vi "Get Plot Metadata.vi"(0 "Model?":bool, 5 "Row Number":i32[](array[numeric]), 7 "Source Location":i32[](array[numeric]), 9 "UVW":i32[](array[numeric]), 11 "Lower Upper":i32[](array[numeric]), 12 "Interation number":i32) -> (1 "Wind Direction":dbl format="%0.2f", 3 "Lower upper":string[][](array[string]), 4 "Locations":string[][](array[string]), 6 "UVW":string[][](array[string]), 8 "Source Locations":string[][](array[string]), 10 "Max Min array":dbl[][](array[numeric]), 13 "Raw Data Filenames":string[](array[string]), 15 "Stl Filename":string)   [LabVIEW 2021]
uses:
  Anemometry/Anemometry Sub Vis/Data_plotting_vis/Results_plotter_Global.vi
  <vilib>/Analysis/NI_AALBase.lvlib
  RFP_Table_Global.vi
  <vilib>/Analysis/baseanly.llb/Mean (DBL).vi
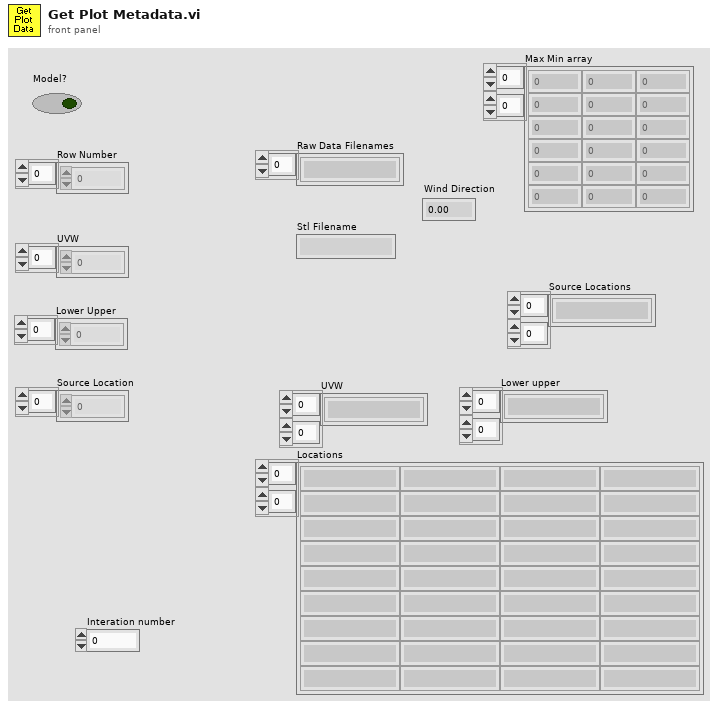
[diagram p1: front panel]
types:
  T1 = enum16{"To Traverse Coordinates", "To User Coordinates"}
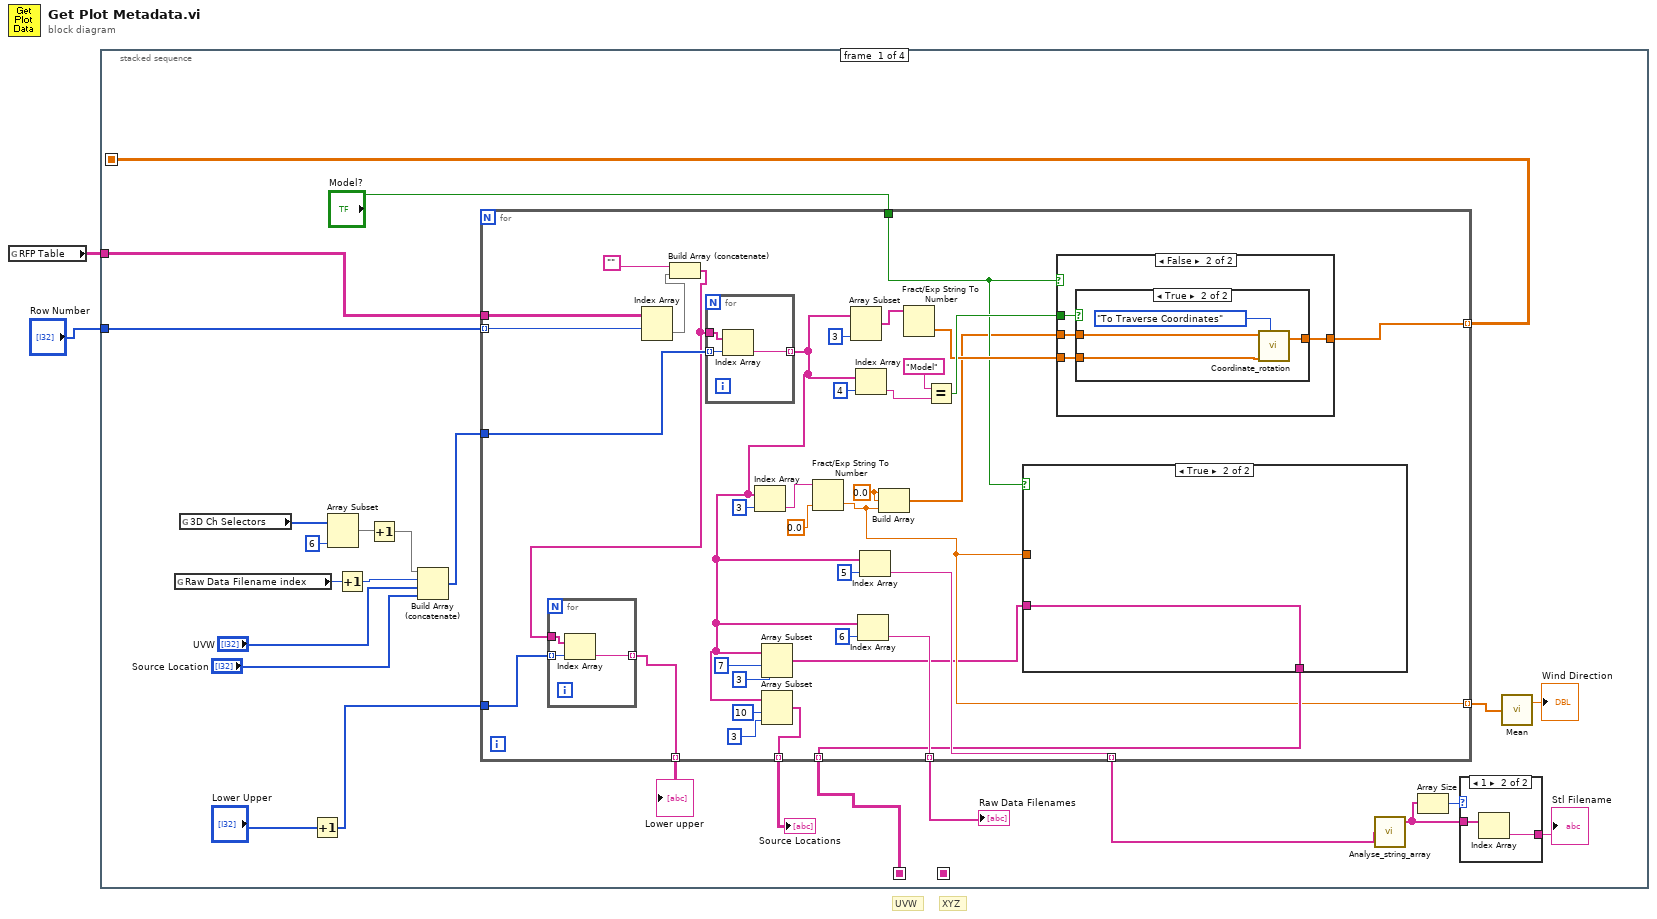
[diagram p0: block diagram]
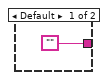
[diagram p2: hidden frame]
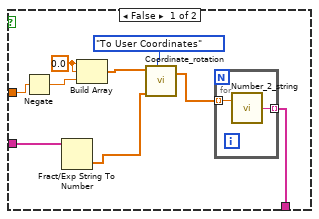
[diagram p3: hidden frame]
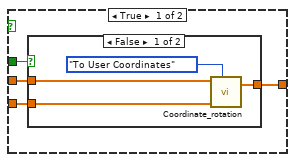
[diagram p4: hidden frame]
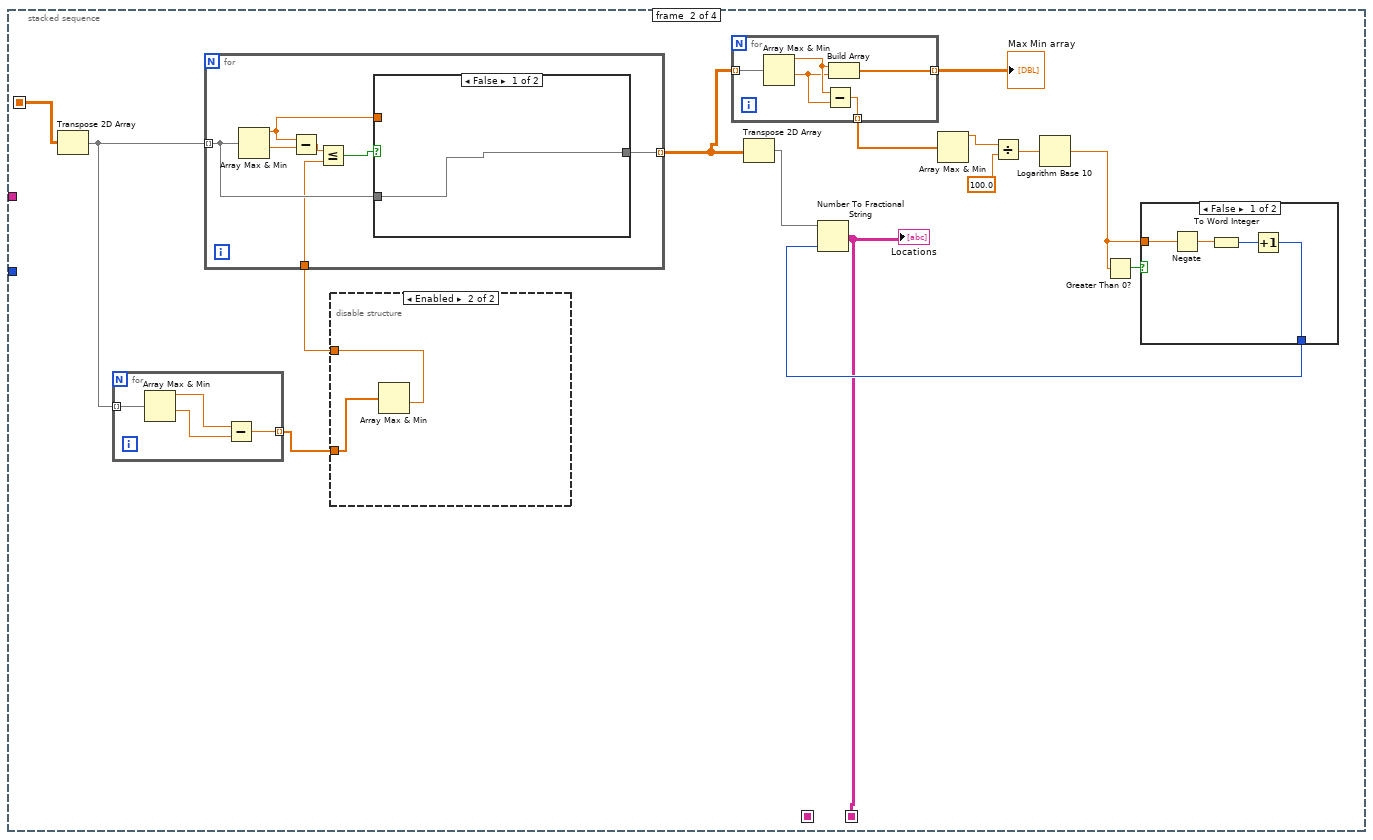
[diagram p7: hidden frame]
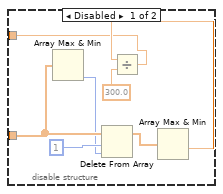
[diagram p8: hidden frame]
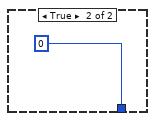
[diagram p9: hidden frame]
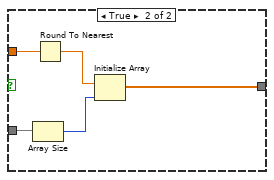
[diagram p10: hidden frame]
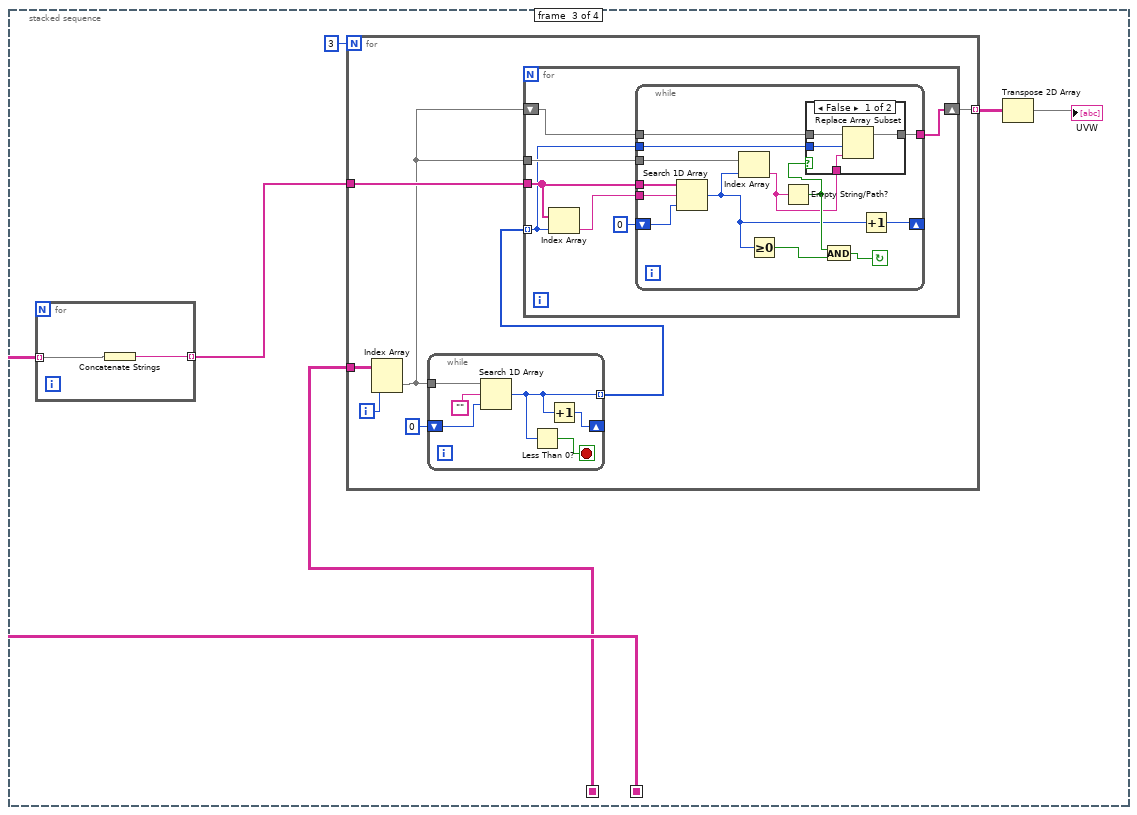
[diagram p11: hidden frame]
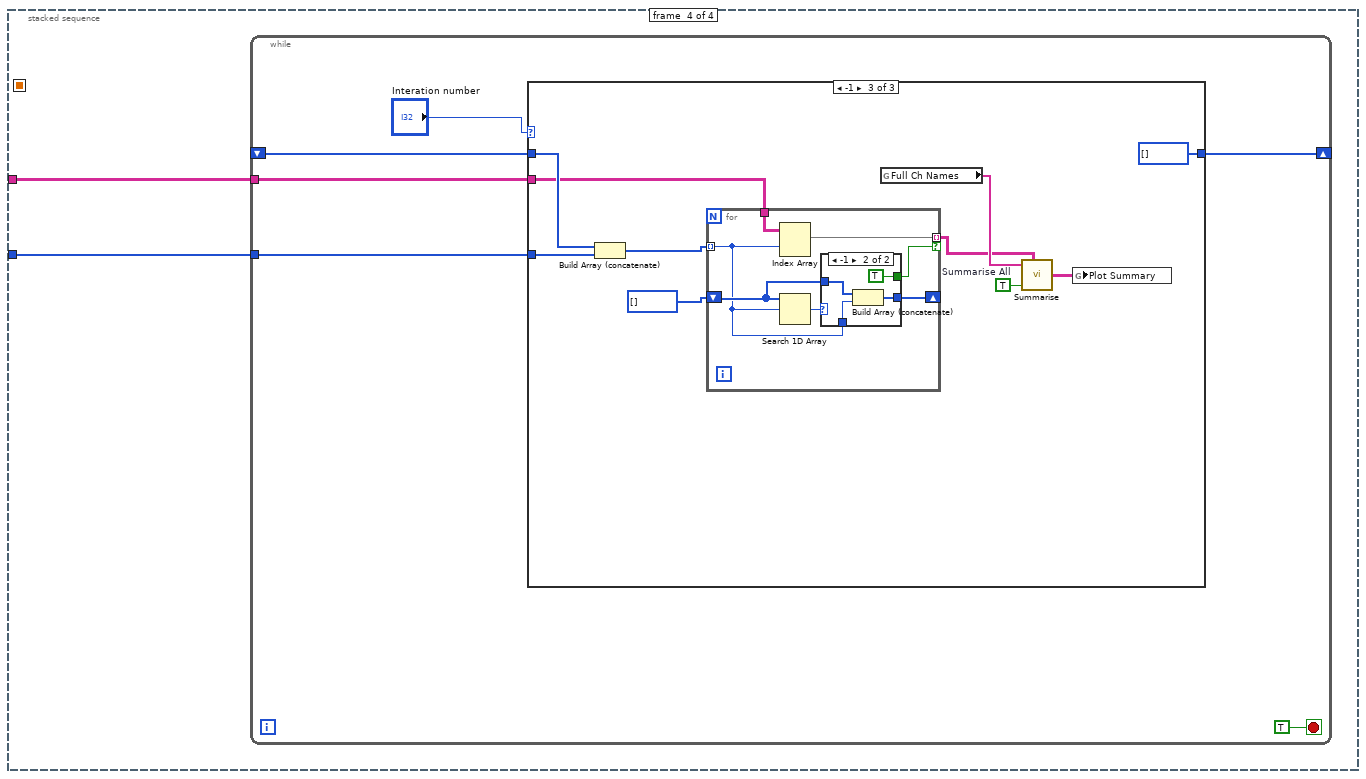
[diagram p13: hidden frame]
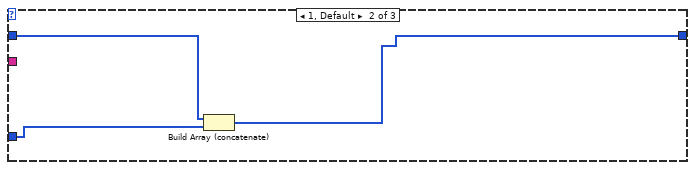
[diagram p15: hidden frame]
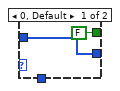
[diagram p16: hidden frame]
diagram:
  # "XYZ"
  # "UVW"
  n1 = global read "RFP_Table_Global.vi" "RFP Table"() -> (w2:string[][])
  n2 = stacked-sequence {
    seq-local: [w24 _ _ _] -> [_ w105 _ _]
    seq-local: [w5 _ _ _] -> [_ _ w156 _]
    seq-local: [_ w102 _ _] -> [_ _ w158 _]
    tunnel: w2 -> [w4 _ _ w199]
    tunnel: "Row Number" -> [w3 _ _ w200]
    frame #0 {
      n3 = global read "Results_plotter_Global.vi" "Raw Data Filename index"() -> (w22:i32)
      n4 = global read "Results_plotter_Global.vi" "3D Ch Selectors"() -> (w26:i32[])
      n5 = Increment(x="Lower Upper") -> (x+1=w11:i32[])
      n6 = Array Subset(array=w26, length=6) -> (w7:i32[])  [unwired: 1 in]
      n7 = Increment(x=w22) -> (x+1=w17:i32)
      n8 = Increment(x=w7) -> (x+1=w6:i32[])
      n9 = Build Array (concatenate)(w6, w17, "UVW", "Source Location") -> (w23:i32[])
      n10 = for {
        tunnel: w3 -> [w65] mode=indexing
        tunnel: w23 -> [w64]
        tunnel: "Model?" -> [w46]
        tunnel: [w54] -> w24 mode=indexing
        tunnel: [w44] -> w5 mode=indexing
        tunnel: [w49] -> w18 mode=indexing
        tunnel: [w47] -> w15 mode=indexing
        tunnel: [w43] -> w14 mode=indexing
        tunnel: w11 -> [w41]
        tunnel: [w40] -> w10 mode=indexing
        tunnel: [w34] -> w8 mode=indexing
        tunnel: w4 -> [w31]
        w57 = 0.0 ("element")
        n11 = Index Array(array=w31, index (row)=w65) -> (element=w51:string[])  [unwired: 1 in]
        n12 = Build Array (concatenate)("", w51) -> (w42:string[])
        n13 = for {
          tunnel: w41 -> [w68] mode=indexing
          tunnel: w42 -> [w67]
          tunnel: [w66] -> w40 mode=indexing
          n14 = Index Array(array=w67, index=w68) -> (element=w66:string)
        }
        n15 = for {
          tunnel: w64 -> [w101] mode=indexing
          tunnel: w42 -> [w100]
          tunnel: [w99] -> w37 mode=indexing
          n16 = Index Array(array=w100, index=w101) -> (element=w99:string)
        }
        n17 = Index Array(array=w37, index=3) -> (element=w56:string)
        n18 = Array Subset(array=w37, index=7, length=3) -> (w38:string[])
        n19 = Array Subset(array=w37, index=10, length=3) -> (w34:string[])
        n20 = Fract/Exp String To Number(string=w56, default (0 dbl)=0.0 ("default (0 DBL)")) -> (number=w43:dbl)  [unwired: 2 in, 1 out]
        n21 = Array Subset(array=w37, length=3) -> (w61:string[])  [unwired: 1 in]
        n22 = Index Array(array=w37, index=4) -> (element=w60:string)
        n23 = Index Array(array=w37, index=6) -> (element=w47:string)
        n24 = Index Array(array=w37, index=5) -> (element=w49:string)
        n25 = Build Array(w57, w57, w43) -> (w45:dbl[])
        n26 = Fract/Exp String To Number(string=w61) -> (number=w53:dbl[])  [unwired: 3 in, 1 out]
        n27 = Equal?(x="Model", y=w60) -> (x = y?=w55:bool)
        n28 = case shown="True" w46 {
          tunnel: [w76 w80] -> w44
          tunnel: w38 -> [w75 w80]
          tunnel: w43 -> [w69 _]
          frame False {
            w72 = 0.0 ("element")
            n29 = Negate(x=w69) -> (-x=w70:dbl)
            n30 = Fract/Exp String To Number(string=w75) -> (number=w74:dbl[])  [unwired: 3 in, 1 out]
            n31 = Build Array(w72, w72, w70) -> (w71:dbl[])
            n32 = call "Coordinate_rotation.vi"("Roll-Pitch-Yaw"=w71, "Input Position"=w74, "Mode"=T1."To User Coordinates") -> ("Output Position"=w73:sgl[])  [unwired: 2 in, 1 out]
            n33 = for {
              tunnel: w73 -> [w79] mode=indexing
              tunnel: [w78] -> w76 mode=indexing
              n34 = call "Number_2_string.vi"("number"=w79) -> ("String"=w78:string)  [unwired: 1 in]
            }
          }
          frame True {
          }
        }
        n35 = case shown="False" w46 {
          tunnel: w55 -> [w84 w93]
          tunnel: [w83 w92] -> w54
          tunnel: w53 -> [w82 w91]
          tunnel: w45 -> [w81 w90]
          frame True {
            n36 = case shown="False" w84 {
              tunnel: [w85 w89] -> w83
              tunnel: w82 -> [w87 w89]
              tunnel: w81 -> [w86 _]
              frame False {
                n37 = call "Coordinate_rotation.vi"("Roll-Pitch-Yaw"=w86, "Input Position"=w87, "Mode"=T1."To User Coordinates") -> ("Output Position"=w85:sgl[])  [unwired: 2 in, 1 out]
              }
              frame True {
              }
            }
          }
          frame False {
            n38 = case shown="True" w93 {
              tunnel: [w94 w97] -> w92
              tunnel: w91 -> [w94 w98]
              tunnel: w90 -> [_ w96]
              frame False {
              }
              frame True {
                n39 = call "Coordinate_rotation.vi"("Roll-Pitch-Yaw"=w96, "Input Position"=w98, "Mode"=T1."To Traverse Coordinates") -> ("Output Position"=w97:sgl[])  [unwired: 2 in, 1 out]
              }
            }
          }
        }
      }
      "Raw Data Filenames" <- w15
      "Lower upper" <- w10
      "Source Locations" <- w8
      n40 = call "Analyse_string_array.vi"("String array"=w18) -> ("Unique strings"=w20:string[])  [unwired: 1 in, 1 out]
      n41 = Array Size(array=w20) -> (size(s)=w21:i32)
      n42 = case shown="1" w21 {
        tunnel: w20 -> [_ w30]
        tunnel: ["" w29] -> w19
        frame Default {
        }
        frame 1 {
          n43 = Index Array(array=w30) -> (element=w29:string)  [unwired: 1 in]
        }
      }
      "Stl Filename" <- w19
      n44 = call-poly <vilib>:"Mean.vi"("X"=w14) -> ("mean"=→"Wind Direction":dbl)  [unwired: 1 out]
    }
    frame #1 {
      n45 = Transpose 2D Array(2D array=w105) -> (transposed array=w106:dbl[][])
      n46 = for {
        tunnel: w106 -> [w129] mode=indexing
        tunnel: [w127] -> w104 mode=indexing
        n47 = Array Max & Min(array=w129) -> (max value=w128:dbl, min value=w126:dbl)  [unwired: 2 out]
        n48 = Subtract(x=w128, y=w126) -> (x-y=w127:dbl)
      }
      n49 = disable-structure shown="Enabled" {
        disable-tunnel: w104 -> [w122 w125]
        disable-tunnel: [w118 w124] -> w103
        frame Disabled {
          n50 = Array Max & Min(array=w122) -> (min index (indices)=w117:i32)  [unwired: 3 out]
          n51 = Delete From Array(array=w122, length=1, index=w117) -> (array with subset deleted=w119:dbl[])  [unwired: 1 out]
          n52 = Array Max & Min(array=w119) -> (min value=w120:dbl)  [unwired: 3 out]
          n53 = Divide(x=w120, y=300.0) -> (x/y=w118:dbl)
        }
        frame Enabled {
          n54 = Array Max & Min(array=w125) -> (min value=w124:dbl)  [unwired: 3 out]
        }
      }
      n55 = for {
        tunnel: w106 -> [w143] mode=indexing
        tunnel: [w142] -> w116 mode=indexing
        tunnel: w103 -> [w141]
        n56 = Array Max & Min(array=w143) -> (max value=w144:dbl, min value=w146:dbl)  [unwired: 2 out]
        n57 = Subtract(x=w144, y=w146) -> (x-y=w145:dbl)
        n58 = Less Or Equal?(x=w145, y=w141) -> (x <= y?=w140:bool)
        n59 = case shown="False" w140 {
          tunnel: w144 -> [_ w152]
          tunnel: w143 -> [w147 w151]
          tunnel: [w147 w148] -> w142
          frame False {
          }
          frame True {
            n60 = Array Size(array=w151) -> (size(s)=w150:i32)
            n61 = Round To Nearest(number=w152) -> (nearest integer value=w149:dbl)
            n62 = Initialize Array(w149, w150) -> (w148:dbl[])
          }
        }
      }
      n63 = for {
        tunnel: w116 -> [w139] mode=indexing
        tunnel: [w138] -> w115 mode=indexing
        tunnel: [w135] -> w113 mode=indexing
        n64 = Array Max & Min(array=w139) -> (max value=w137:dbl, min value=w136:dbl)  [unwired: 2 out]
        n65 = Subtract(x=w137, y=w136) -> (x-y=w135:dbl)
        n66 = Build Array(w137, w136) -> (w138:dbl[])
      }
      "Max Min array" <- w115
      n67 = Transpose 2D Array(2D array=w116) -> (transposed array=w114:dbl[][])
      n68 = Array Max & Min(array=w113) -> (max value=w112:dbl)  [unwired: 3 out]
      n69 = Divide(x=w112, y=100.0) -> (x/y=w110:dbl)
      n70 = Logarithm Base 10(1:w110) -> (0:w108:dbl)
      n71 = Greater Than 0?(x=w108) -> (x > 0?=w109:bool)
      n72 = case shown="False" w109 {
        tunnel: w108 -> [w133 _]
        tunnel: [w130 i16 0 ("precision (6)")] -> w107
        frame False {
          n73 = Negate(x=w133) -> (-x=w132:dbl)
          n74 = To Word Integer(number=w132) -> (16bit integer=w131:i16)
          n75 = Increment(x=w131) -> (x+1=w130:i16)
        }
        frame True {
        }
      }
      n76 = Number To Fractional String(number=w114, precision (6)=w107) -> (F-format string=w102:string[][])  [unwired: 2 in]
      "Locations" <- w102
    }
    frame #2 {
      n77 = for {
        tunnel: w158 -> [w198] mode=indexing
        tunnel: [w197] -> w157 mode=indexing
        n78 = Concatenate Strings(w198) -> (w197:string)
      }
      n79 = for {
        N: 3 -> [_]
        tunnel: w157 -> [w161]
        tunnel: w156 -> [w165]
        tunnel: [w159] -> w154 mode=indexing
        i -> [w164]
        n80 = Index Array(array=w165, index (col)=w164) -> (element=w160:string[])  [unwired: 1 in]
        n81 = while {
          tunnel: w160 -> [w171]
          shift-right: [w166] -> _
          shift-left: 0 ("index of element") -> [w169]
          tunnel: [w167] -> w162 mode=indexing
          stop <- w168 stop-if-true
          n82 = Search 1D Array(1D array=w171, element="", start index (0)=w169) -> (index of element=w167:i32)
          n83 = Less Than 0?(x=w167) -> (x < 0?=w168:bool)
          n84 = Increment(x=w167) -> (x+1=w166:i32)
        }
        n85 = for {
          tunnel: w161 -> [w178]
          tunnel: w162 -> [w172] mode=indexing
          tunnel: w160 -> [w175]
          shift-right: [w173] -> w159
          shift-left: w160 -> [w174]
          n86 = Index Array(array=w178, index=w172) -> (element=w177:string)
          n87 = while {
            tunnel: w178 -> [w191]
            tunnel: w177 -> [w190]
            shift-right: [w179] -> _
            shift-left: 0 ("index of element") -> [w189]
            tunnel: w175 -> [w188]
            tunnel: w174 -> [w184]
            tunnel: [w183] -> w173
            tunnel: w172 -> [w181]
            stop <- w186 continue-if-true
            n88 = Search 1D Array(1D array=w191, element=w190, start index (0)=w189) -> (index of element=w180:i32)
            n89 = Index Array(array=w188, index=w180) -> (element=w182:string)
            n90 = Greater Or Equal To 0?(x=w180) -> (x >= 0?=w187:bool)
            n91 = Empty String/Path?(string/path=w182) -> (empty?=w185:bool)
            n92 = case shown="False" w185 {
              tunnel: w184 -> [w195 w196]
              tunnel: [w194 w196] -> w183
              tunnel: w181 -> [w193 _]
              tunnel: w182 -> [w192 _]
              frame False {
                n93 = Replace Array Subset(array=w195, new element=w192, index=w193) -> (w194:string[])
              }
              frame True {
              }
            }
            n94 = And(x=w185, y=w187) -> (x .and. y?=w186:bool)
            n95 = Increment(x=w180) -> (x+1=w179:i32)
          }
        }
      }
      n96 = Transpose 2D Array(2D array=w154) -> (transposed array=→"UVW":string[][])
    }
    frame #3 {
      n97 = while {
        shift-right: [w205] -> _
        shift-left: _ -> [w203]
        tunnel: w200 -> [w204]
        tunnel: w199 -> [w201]
        stop <- TRUE stop-if-true
        n98 = case shown="-1" "Interation number" {
          tunnel: [w207 w208 i32[] [] ("Row Number")] -> w205
          tunnel: w204 -> [w207 w210 w220]
          tunnel: w203 -> [_ w209 w219]
          tunnel: w201 -> [_ _ w216]
          frame 0 {
          }
          frame 1, Default {
            n99 = Build Array (concatenate)(w209, w210) -> (w208:i32[])
          }
          frame -1 {
            w218 = TRUE  # Summarise All
            n100 = Build Array (concatenate)(w219, w220) -> (w215:i32[])
            n101 = for {
              tunnel: w216 -> [w227]
              tunnel: [w226] -> w212 mode=indexing if=w222
              tunnel: w215 -> [w221] mode=indexing
              shift-right: [w224] -> _
              shift-left: i32[] [] -> [w223]
              n102 = Index Array(array=w227, index (row)=w221) -> (element=w226:string[])  [unwired: 1 in]
              n103 = Search 1D Array(1D array=w223, element=w221) -> (index of element=w225:i32)  [unwired: 1 out]
              n104 = case shown="-1" w225 {
                tunnel: w221 -> [_ w233]
                tunnel: w223 -> [w229 w232]
                tunnel: [w229 w231] -> w224
                tunnel: [FALSE TRUE] -> w222
                frame 0, Default {
                }
                frame -1 {
                  n105 = Build Array (concatenate)(w232, w233) -> (w231:i32[])
                }
              }
            }
            n106 = global read "Results_plotter_Global.vi" "Full Ch Names"() -> (w213:string[])
            n107 = call "Summarise.vi"("Channel Names"=w213, "Data"=w212, "Summarise All"=w218) -> ("Summary"=w217:string[][])  [unwired: 2 in]
            n108 = global write "Results_plotter_Global.vi" "Plot Summary"(w217) -> ()
          }
        }
      }
    }
  }
